vi "Go To Magnet Field.vi"(6 "Persistent at Target Field?":bool, 8 "error in (no error)":errorcluster, 9 "Target Field Rate (T/min)":dbl, 10 "Target Field (T)":dbl, 11 "instrument.PPMS2 in":refnum<class "instrument.PPMS2.lvclass">) -> (0 "error out":errorcluster, 3 "instrument.PPMS2 out":refnum<class "instrument.PPMS2.lvclass">)   [LabVIEW 2016, in "instrument.PPMS2.lvclass"]
uses:
  instrument.PPMS2.lvclass
  PPMS Global.vi
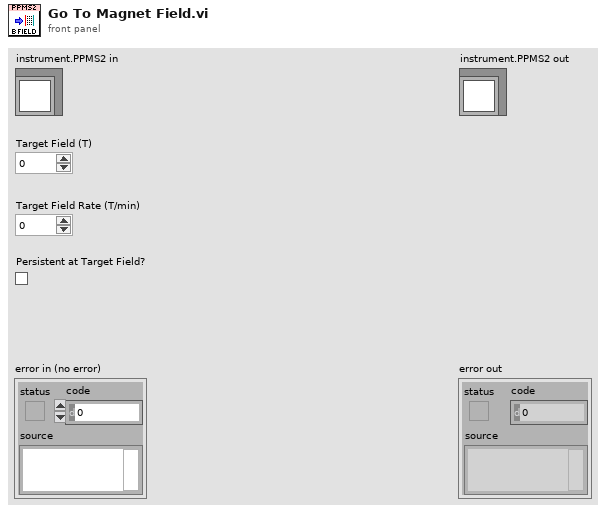
[diagram p1: front panel]
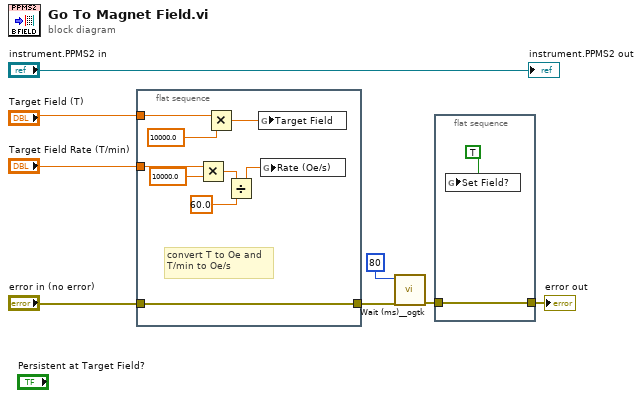
[diagram p0: block diagram]
diagram:
  n1 = flat-sequence {
    tunnel: "error in (no error)" -> [w17]
    tunnel: [w17] -> w3
    tunnel: "Target Field (T)" -> [w16]
    tunnel: "Target Field Rate (T/min)" -> [w13]
    frame #0 {
      # "convert T to Oe and\nT/min to Oe/s"
      n2 = Multiply(x=w13, y=10000.0) -> (x*y=w12:dbl)
      n3 = Multiply(x=w16, y=10000.0) -> (x*y=w15:dbl)
      n4 = Divide(x=w12, y=60.0) -> (x/y=w10:dbl)
      n5 = global write "PPMS Global.vi" "Target Field"(w15) -> ()
      n6 = global write "PPMS Global.vi" "Rate (Oe/s)"(w10) -> ()
    }
  }
  n7 = call <userlib>:"Wait (ms)__ogtk.vi"("error in (no error)"=w3, "milliseconds to wait"=u32 80) -> ("error out"=w7:errorcluster)  [unwired: 8 in, 1 out]
  n8 = flat-sequence {
    tunnel: w7 -> [w18]
    tunnel: [w18] -> w6
    frame #0 {
      n9 = global write "PPMS Global.vi" "Set Field?"(TRUE ("Set Field?")) -> ()
    }
  }
  "error out" <- w6
  "instrument.PPMS2 out" <- "instrument.PPMS2 in"
